vi "test_read-nmea-data2.vi"() -> ()   [LabVIEW 2019] (continued)
15:15:18.22\tF9P\t\t\n15:15:18.24\tF9P\t$GNRMC,061520.00,A,3723.59873,N,12656.93743,E,2.458,246.74,250720,,,A,V*09\n\t\n15:15:18.26\tF9P\t$GNVTG,246.74,T,,M,2.458,N,4.552,K,A*2D\n\t\n15:15:18.28\tF9P\t$GNGGA,061520.00,3723.59873,N,12656.93743,E,1,12,0.71,46.1,M,18.5,M,,*71\n\t\n15:15:18.30\tF9P\t$GNGSA,A,3,12,06,19,05,17,09,04,02,,,,,1.21,0.71,0.98,1*05\n\t\n15:15:18.32\tF9P\t$GNGSA,A,3,85,70,71,84,,,,,,,,,1.21,0.71,0.98,2*07\n\t\n15:15:18.34\tF9P\t$GNGSA,A,3,36,19,11,04,09,12,,,,,,,1.21,0.71,0.98,3*05\n\t\n15:15:18.36\tF9P\t$GNGSA,A,3,14,11,33,,,,,,,,,,1.21,0.71,0.98,4*04\n\t\n15:15:18.38\tF9P\t$GPGSV,3,1,09,02,56,320,31,04,17,043,28,05,38,248,31,06,64,051,27,1*65\n\t\n15:15:18.40\tF9P\t$GPGSV,3,2,09,09,44,072,41,12,23,275,26,17,31,154,27,19,51,157,28,1*67\n\t\n15:15:18.42\tF9P\t$GPGSV,3,3,09,25,12,305,21,1*5C\n\t\n15:15:18.44\tF9P\t$GPGSV,3,1,09,02,56,320,,04,17,043,22,05,38,248,31,06,64,051,29,6*64\n\t\n15:15:18.46\tF9P\t$GPGSV,3,2,09,09,44,072,34,12,23,275,18,17,31,154,20,19,51,157,,6*62\n\t\n15:15:18.48\tF9P\t$GPGSV,3,3,09,25,12,305,,6*58\n\t\n15:15:18.50\tF9P\t$GLGSV,2,1,08,69,10,031,27,70,70,037,28,71,54,207,33,72,05,210,,1*75\n\t\n15:15:18.52\tF9P\t$GLGSV,2,2,08,77,01,324,,84,19,123,16,85,69,072,38,86,38,331,,1*7F\n\t\n15:15:18.54\tF9P\t$GLGSV,2,1,08,69,10,031,20,70,70,037,,71,54,207,24,72,05,210,,3*7C\n\t\n15:15:18.56\tF9P\t$GLGSV,2,2,08,77,01,324,,84,19,123,20,85,69,072,26,86,38,331,,3*77\n\t\n15:15:18.58\tF9P\t$GAGSV,2,1,08,02,08,296,11,04,67,114,38,09,33,193,29,11,72,001,24,7*7E\n\t\n15:15:18.60\tF9P\t$GAGSV,2,2,08,12,39,103,24,19,25,045,30,25,08,248,,36,27,309,22,7*70\n\t\n15:15:18.62\tF9P\t$GAGSV,2,1,08,02,08,296,,04,67,114,,09,33,193,21,11,72,001,,2*7E\n\t\n15:15:18.64\tF9P\t$GAGSV,2,2,08,12,39,103,,19,25,045,22,25,08,248,,36,27,309,19,2*78\n\t\n15:15:18.66\tF9P\t$GBGSV,2,1,06,07,,,24,11,48,133,27,14,87,101,28,28,,,26,1*74\n\t\n15:15:18.68\tF9P\t$GBGSV,2,2,06,33,62,220,32,34,,,32,1*43\n\t\n15:15:18.70\tF9P\t$GBGSV,1,1,03,11,48,133,25,14,87,101,29,33,62,220,,3*48\n\t\n15:15:18.72\tF9P\t$GNGLL,3723.59873,N,12656.93743,E,061520.00,A,A*7E\n\t\n15:15:18.74\tF9P\t\t\n15:15:18.76\tF9P\t\t\n15:15:18.78\tF9P\t\t\n15:15:18.80\tF9P\t\t\n15:15:18.82\tF9P\t\t\n15:15:18.84\tF9P\t\t\n15:15:18.86\tF9P\t\t\n15:15:18.88\tF9P\t\t\n15:15:18.90\tF9P\t\t\n15:15:18.92\tF9P\t\t\n15:15:18.94\tF9P\t\t\n15:15:18.96\tF9P\t\t\n15:15:18.98\tF9P\t\t\n15:15:19.00\tF9P\t\t\n15:15:19.02\tF9P\t\t\n15:15:19.04\tF9P\t\t\n15:15:19.06\tF9P\t\t\n15:15:19.08\tF9P\t\t\n15:15:19.10\tF9P\t\t\n15:15:19.12\tF9P\t\t\n15:15:19.14\tF9P\t\t\n15:15:19.16\tF9P\t\t\n15:15:19.18\tF9P\t\t\n15:15:19.20\tF9P\t\t\n15:15:19.22\tF9P\t\t\n15:15:19.24\tF9P\t$GNRMC,061521.00,A,3723.59850,N,12656.93661,E,2.546,240.41,250720,,,A,V*06\n\t\n15:15:19.26\tF9P\t$GNVTG,240.41,T,,M,2.546,N,4.715,K,A*22\n\t\n15:15:19.28\tF9P\t$GNGGA,061521.00,3723.59850,N,12656.93661,E,1,12,0.68,46.5,M,18.5,M,,*7C\n\t\n15:15:19.30\tF9P\t$GNGSA,A,3,12,06,19,05,17,09,04,02,,,,,1.19,0.68,0.98,1*06\n\t\n15:15:19.32\tF9P\t$GNGSA,A,3,85,70,71,84,,,,,,,,,1.19,0.68,0.98,2*04\n\t\n15:15:19.34\tF9P\t$GNGSA,A,3,36,19,11,04,09,12,,,,,,,1.19,0.68,0.98,3*06\n\t\n15:15:19.36\tF9P\t$GNGSA,A,3,14,11,33,,,,,,,,,,1.19,0.68,0.98,4*07\n\t\n15:15:19.38\tF9P\t$GPGSV,3,1,09,02,56,320,25,04,17,043,27,05,38,248,30,06,64,051,26,1*6F\n\t\n15:15:19.40\tF9P\t$GPGSV,3,2,09,09,44,072,43,12,23,275,35,17,31,154,28,19,51,157,28,1*68\n\t\n15:15:19.42\tF9P\t$GPGSV,3,3,09,25,12,305,20,1*5D\n\t\n15:15:19.44\tF9P\t$GPGSV,3,1,09,02,56,320,,04,17,043,21,05,38,248,22,06,64,051,29,6*65\n\t\n15:15:19.46\tF9P\t$GPGSV,3,2,09,09,44,072,31,12,23,275,18,17,31,154,18,19,51,157,,6*6C\n\t\n15:15:19.48\tF9P\t$GPGSV,3,3,09,25,12,305,,6*58\n\t\n15:15:19.50\tF9P\t$GLGSV,2,1,08,69,10,031,25,70,70,037,29,71,54,207,37,72,05,210,,1*72\n\t\n15:15:19.52\tF9P\t$GLGSV,2,2,08,77,01,324,,84,19,123,14,85,69,072,37,86,38,331,,1*72\n\t\n15:15:19.54\tF9P\t$GLGSV,2,1,08,69,10,031,19,70,70,037,,71,54,207,25,72,05,210,,3*77\n\t\n15:15:19.56\tF9P\t$GLGSV,2,2,08,77,01,324,,84,19,123,20,85,69,072,26,86,38,331,,3*77\n\t\n15:15:19.58\tF9P\t$GAGSV,2,1,08,02,08,296,10,04,67,114,39,09,33,193,35,11,72,001,24,7*73\n\t\n15:15:19.60\tF9P\t$GAGSV,2,2,08,12,39,103,24,19,25,045,28,25,08,248,,36,27,309,23,7*78\n\t\n15:15:19.62\tF9P\t$GAGSV,2,1,08,02,08,296,,04,67,114,,09,33,193,20,11,72,001,,2*7F\n\t\n15:15:19.64\tF9P\t$GAGSV,2,2,08,12,39,103,,19,25,045,22,25,08,248,,36,27,309,18,2*79\n\t\n15:15:19.66\tF9P\t$GBGSV,2,1,06,07,,,24,11,48,133,28,14,87,101,32,28,,,26,1*70\n\t\n15:15:19.68\tF9P\t$GBGSV,2,2,06,33,62,220,33,34,,,26,1*47\n\t\n15:15:19.70\tF9P\t$GBGSV,1,1,03,11,48,133,,14,87,101,,33,62,220,,3*44\n\t\n15:15:19.72\tF9P\t$GNGLL,3723.59850,N,12656.93661,E,061521.00,A,A*7F\n\t\n15:15:19.74\tF9P\t\t\n15:15:19.76\tF9P\t\t\n15:15:19.78\tF9P\t\t\n15:15:19.80\tF9P\t\t\n15:15:19.82\tF9P\t\t\n15:15:19.84\tF9P\t\t\n15:15:19.86\tF9P\t\t\n15:15:19.88\tF9P\t\t\n15:15:19.90\tF9P\t\t\n15:15:19.92\tF9P\t\t\n15:15:19.94\tF9P\t\t\n15:15:19.96\tF9P\t\t\n15:15:19.98\tF9P\t\t\n15:15:20.00\tF9P\t\t\n15:15:20.02\tF9P\t\t\n15:15:20.04\tF9P\t\t\n15:15:20.06\tF9P\t\t\n15:15:20.08\tF9P\t\t\n15:15:20.10\tF9P\t\t\n15:15:20.12\tF9P\t\t\n15:15:20.14\tF9P\t\t\n15:15:20.16\tF9P\t\t\n15:15:20.18\tF9P\t\t\n15:15:20.20\tF9P\t\t\n15:15:20.22\tF9P\t\t\n15:15:20.24\tF9P\t$GNRMC,061522.00,A,3723.59832,N,12656.93567,E,2.630,241.81,250720,,,A,V*0B\n\t\n15:15:20.26\tF9P\t$GNVTG,241.81,T,,M,2.630,N,4.870,K,A*21\n\t\n15:15:20.28\tF9P\t$GNGGA,061522.00,3723.59832,N,12656.93567,E,1,12,0.65,46.4,M,18.5,M,,*72\n\t\n15:15:20.30\tF9P\t$GNGSA,A,3,12,06,19,05,17,09,04,02,,,,,1.15,0.65,0.95,1*0A\n\t\n15:15:20.32\tF9P\t$GNGSA,A,3,85,70,71,84,,,,,,,,,1.15,0.65,0.95,2*08\n\t\n15:15:20.34\tF9P\t$GNGSA,A,3,36,19,11,04,09,12,,,,,,,1.15,0.65,0.95,3*0A\n\t\n15:15:20.36\tF9P\t$GNGSA,A,3,14,11,33,,,,,,,,,,1.15,0.65,0.95,4*0B\n\t\n15:15:20.38\tF9P\t$GPGSV,3,1,09,02,56,320,31,04,17,043,38,05,38,248,29,06,64,051,31,1*6A\n\t\n15:15:20.40\tF9P\t$GPGSV,3,2,09,09,44,072,40,12,23,275,32,17,31,154,29,19,51,157,28,1*6D\n\t\n15:15:20.42\tF9P\t$GPGSV,3,3,09,25,12,305,19,1*57\n\t\n15:15:20.44\tF9P\t$GPGSV,3,1,09,02,56,320,,04,17,043,21,05,38,248,22,06,64,051,28,6*64\n\t\n15:15:20.46\tF9P\t$GPGSV,3,2,09,09,44,072,26,12,23,275,18,17,31,154,19,19,51,157,,6*6B\n\t\n15:15:20.48\tF9P\t$GPGSV,3,3,09,25,12,305,,6*58\n\t\n15:15:20.50\tF9P\t$GLGSV,2,1,08,69,10,031,25,70,70,037,24,71,54,207,29,72,05,210,,1*70\n\t\n15:15:20.52\tF9P\t$GLGSV,2,2,08,77,01,324,,84,19,123,14,85,69,072,35,86,38,331,,1*70\n\t\n15:15:20.54\tF9P\t$GLGSV,2,1,08,69,10,031,18,70,70,037,,71,54,207,30,72,05,210,,3*72\n\t\n15:15:20.56\tF9P\t$GLGSV,2,2,08,77,01,324,,84,19,123,20,85,69,072,26,86,38,331,,3*77\n\t\n15:15:20.58\tF9P\t$GAGSV,2,1,08,02,08,296,13,04,67,114,36,09,33,193,26,11,72,001,25,7*7C\n\t\n15:15:20.60\tF9P\t$GAGSV,2,2,08,12,39,103,25,19,25,045,29,25,08,248,,36,27,309,23,7*78\n\t\n15:15:20.62\tF9P\t$GAGSV,2,1,08,02,08,296,,04,67,114,,09,33,193,20,11,72,001,,2*7F\n\t\n15:15:20.64\tF9P\t$GAGSV,2,2,08,12,39,103,,19,25,045,21,25,08,248,,36,27,309,20,2*71\n\t\n15:15:20.66\tF9P\t$GBGSV,2,1,06,07,,,29,11,48,133,26,14,87,101,29,28,,,25,1*7A\n\t\n15:15:20.68\tF9P\t$GBGSV,2,2,06,33,62,220,38,34,,,25,1*4F\n\t\n15:15:20.70\tF9P\t$GBGSV,1,1,03,11,48,133,,14,87,101,,33,62,220,,3*44\n\t\n15:15:20.72\tF9P\t$GNGLL,3723.59832,N,12656.93567,E,061522.00,A,A*7D\n\t\n15:15:20.74\tF9P\t\t\n15:15:20.76\tF9P\t\t\n15:15:20.78\tF9P\t\t\n15:15:20.80\tF9P\t\t\n15:15:20.82\tF9P\t\t\n15:15:20.84\tF9P\t\t\n15:15:20.86\tF9P\t\t\n15:15:20.88\tF9P\t\t\n15:15:20.90\tF9P\t\t\n15:15:20.92\tF9P\t\t\n15:15:20.94\tF9P\t\t\n15:15:20.96\tF9P\t\t\n15:15:20.98\tF9P\t\t\n15:15:21.00\tF9P\t\t\n15:15:21.02\tF9P\t\t\n15:15:21.04\tF9P\t\t\n15:15:21.06\tF9P\t\t\n15:15:21.08\tF9P\t\t\n15:15:21.10\tF9P\t\t\n15:15:21.12\tF9P\t\t\n15:15:21.14\tF9P\t\t\n15:15:21.16\tF9P\t\t\n15:15:21.18\tF9P\t\t\n15:15:21.20\tF9P\t\t\n15:15:21.22\tF9P\t\t\n15:15:21.24\tF9P\t$GNRMC,061523.00,A,3723.59801,N,12656.93492,E,2.349,237.20,250720,,,A,V*00\n\t\n15:15:21.26\tF9P\t$GNVTG,237.20,T,,M,2.349,N,4.350,K,A*29\n\t\n15:15:21.29\tF9P\t$GNGGA,061523.00,3723.59801,N,12656.93492,E,1,12,0.69,46.6,M,18.5,M,,*76\n\t\n15:15:21.31\tF9P\t$GNGSA,A,3,12,06,19,05,17,09,04,02,,,,,1.20,0.69,0.98,1*0D\n\t\n15:15:21.33\tF9P\t$GNGSA,A,3,85,70,71,84,,,,,,,,,1.20,0.69,0.98,2*0F\n\t\n15:15:21.35\tF9P\t$GNGSA,A,3,36,19,11,04,09,12,,,,,,,1.20,0.69,0.98,3*0D\n\t\n15:15:21.37\tF9P\t$GNGSA,A,3,14,11,33,,,,,,,,,,1.20,0.69,0.98,4*0C\n\t\n15:15:21.39\tF9P\t$GPGSV,3,1,09,02,56,320,25,04,17,043,35,05,38,248,31,06,64,051,31,1*6B\n\t\n15:15:21.41\tF9P\t$GPGSV,3,2,09,09,44,072,42,12,23,275,31,17,31,154,28,19,51,157,27,1*62\n\t\n15:15:21.43\tF9P\t$GPGSV,3,3,09,25,12,305,18,1*56\n\t\n15:15:21.45\tF9P\t$GPGSV,3,1,09,02,56,320,,04,17,043,20,05,38,248,21,06,64,051,28,6*66\n\t\n15:15:21.47\tF9P\t$GPGSV,3,2,09,09,44,072,31,12,23,275,20,17,31,154,18,19,51,157,,6*67\n\t\n15:15:21.49\tF9P\t$GPGSV,3,3,09,25,12,305,,6*58\n\t\n15:15:21.51\tF9P\t$GLGSV,2,1,08,69,10,031,31,70,70,037,30,71,54,207,31,72,05,210,,1*79\n\t\n15:15:21.53\tF9P\t$GLGSV,2,2,08,77,01,324,,84,19,123,15,85,69,072,38,86,38,331,,1*7C\n\t\n15:15:21.55\tF9P\t$GLGSV,2,1,08,69,10,031,18,70,70,037,,71,54,207,24,72,05,210,,3*77\n\t\n15:15:21.57\tF9P\t$GLGSV,2,2,08,77,01,324,,84,19,123,21,85,69,072,25,86,38,331,,3*75\n\t\n15:15:21.59\tF9P\t$GAGSV,2,1,08,02,08,296,15,04,67,114,32,09,33,193,27,11,72,001,24,7*7E\n\t\n15:15:21.61\tF9P\t$GAGSV,2,2,08,12,39,103,26,19,25,045,29,25,08,248,,36,27,309,23,7*7B\n\t\n15:15:21.63\tF9P\t$GAGSV,2,1,08,02,08,296,,04,67,114,,09,33,193,22,11,72,001,,2*7D\n\t\n15:15:21.65\tF9P\t$GAGSV,2,2,08,12,39,103,,19,25,045,21,25,08,248,,36,27,309,,2*73\n\t\n15:15:21.67\tF9P\t$GBGSV,2,1,06,07,,,24,11,48,133,27,14,87,101,37,28,,,25,1*79\n\t\n15:15:21.69\tF9P\t$GBGSV,2,2,06,33,62,220,38,34,,,24,1*4E\n\t\n15:15:21.71\tF9P\t$GBGSV,1,1,03,11,48,133,,14,87,101,,33,62,220,,3*44\n\t\n15:15:21.73\tF9P\t$GNGLL,3723.59801,N,12656.93492,E,061523.00,A,A*77\n\t\n15:15:21.75\tF9P\t\t\n15:15:21.77\tF9P\t\t\n15:15:21.79\tF9P\t\t\n15:15:21.81\tF9P\t\t\n15:15:21.83\tF9P\t\t\n15:15:21.85\tF9P\t\t\n15:15:21.87\tF9P\t\t\n15:15:21.89\tF9P\t\t\n15:15:21.91\tF9P\t\t\n15:15:21.93\tF9P\t\t\n15:15:21.95\tF9P\t\t\n15:15:21.97\tF9P\t\t\n15:15:21.99\tF9P\t\t\n15:15:22.01\tF9P\t\t\n15:15:22.03\tF9P\t\t\n15:15:22.05\tF9P\t\t\n15:15:22.07\tF9P\t\t\n15:15:22.09\tF9P\t\t\n15:15:22.11\tF9P\t\t\n15:15:22.13\tF9P\t\t\n15:15:22.15\tF9P\t\t\n15:15:22.17\tF9P\t\t\n15:15:22.19\tF9P\t\t\n15:15:22.21\tF9P\t\t\n15:15:22.23\tF9P\t$GNRMC,061524.00,A,3723.59778,N,12656.93396,E,2.598,237.74,250720,,,A,V*0E\n\t\n15:15:22.25\tF9P\t$GNVTG,237.74,T,,M,2.598,N,4.811,K,A*2C\n\t\n15:15:22.27\tF9P\t$GNGGA,061524.00,3723.59778,N,12656.93396,E,1,12,0.71,46.5,M,18.5,M,,*79\n\t\n15:15:22.29\tF9P\t$GNGSA,A,3,12,06,19,05,17,09,04,02,,,,,1.21,0.71,0.98,1*05\n\t\n15:15:22.31\tF9P\t$GNGSA,A,3,85,70,71,84,,,,,,,,,1.21,0.71,0.98,2*07\n\t\n15:15:22.33\tF9P\t$GNGSA,A,3,36,19,11,04,09,12,,,,,,,1.21,0.71,0.98,3*05\n\t\n15:15:22.35\tF9P\t$GNGSA,A,3,14,11,33,,,,,,,,,,1.21,0.71,0.98,4*04\n\t\n15:15:22.37\tF9P\t$GPGSV,3,1,09,02,56,320,31,04,17,043,27,05,38,248,30,06,64,051,36,1*6B\n\t\n15:15:22.39\tF9P\t$GPGSV,3,2,09,09,44,072,26,12,23,275,36,17,31,154,26,19,51,157,27,1*69\n\t\n15:15:22.41\tF9P\t$GPGSV,3,3,09,25,12,305,19,1*57\n\t\n15:15:22.43\tF9P\t$GPGSV,3,1,09,02,56,320,,04,17,043,20,05,38,248,21,06,64,051,27,6*69\n\t\n15:15:22.45\tF9P\t$GPGSV,3,2,09,09,44,072,26,12,23,275,28,17,31,154,17,19,51,157,,6*66\n\t\n15:15:22.47\tF9P\t$GPGSV,3,3,09,25,12,305,,6*58\n\t\n15:15:22.49\tF9P\t$GLGSV,2,1,08,69,10,031,25,70,70,037,25,71,54,207,31,72,05,210,,1*78\n\t\n15:15:22.51\tF9P\t$GLGSV,2,2,08,77,01,324,,84,19,123,15,85,69,072,36,86,38,331,,1*72\n\t\n15:15:22.53\tF9P\t$GLGSV,2,1,08,69,10,031,17,70,70,037,,71,54,207,24,72,05,210,,3*78\n\t\n15:15:22.55\tF9P\t$GLGSV,2,2,08,77,01,324,,84,19,123,21,85,69,072,31,86,38,331,,3*70\n\t\n15:15:22.57\tF9P\t$GAGSV,2,1,08,02,08,296,11,04,67,114,35,09,33,193,27,11,72,002,25,7*7F\n\t\n15:15:22.59\tF9P\t$GAGSV,2,2,08,12,39,103,25,19,25,045,33,25,08,248,,36,27,309,27,7*77\n\t\n15:15:22.61\tF9P\t$GAGSV,2,1,08,02,08,296,,04,67,114,,09,33,193,30,11,72,002,,2*7D\n\t\n15:15:22.63\tF9P\t$GAGSV,2,2,08,12,39,103,,19,25,045,22,25,08,248,,36,27,309,,2*70\n\t\n15:15:22.65\tF9P\t$GBGSV,2,1,06,07,,,23,11,48,133,40,14,87,101,38,28,,,25,1*70\n\t\n15:15:22.67\tF9P\t$GBGSV,2,2,06,33,62,220,35,34,,,31,1*47\n\t\n15:15:22.69\tF9P\t$GBGSV,1,1,03,11,48,133,,14,87,101,,33,62,220,,3*44\n\t\n15:15:22.71\tF9P\t$GNGLL,3723.59778,N,12656.93396,E,061524.00,A,A*72\n\t\n15:15:22.73\tF9P\t\t\n15:15:22.75\tF9P\t\t\n15:15:22.77\tF9P\t\t\n15:15:22.79\tF9P\t\t\n15:15:22.81\tF9P\t\t\n15:15:22.83\tF9P\t\t\n15:15:22.85\tF9P\t\t\n15:15:22.87\tF9P\t\t\n15:15:22.89\tF9P\t\t\n15:15:22.91\tF9P\t\t\n15:15:22.93\tF9P\t\t\n15:15:22.95\tF9P\t\t\n15:15:22.97\tF9P\t\t\n15:15:22.99\tF9P\t\t\n15:15:23.01\tF9P\t\t\n15:15:23.03\tF9P\t\t\n15:15:23.05\tF9P\t\t\n15:15:23.07\tF9P\t\t\n15:15:23.09\tF9P\t\t\n15:15:23.11\tF9P\t\t\n15:15:23.13\tF9P\t\t\n15:15:23.15\tF9P\t\t\n15:15:23.17\tF9P\t\t\n15:15:23.19\tF9P\t\t\n15:15:23.21\tF9P\t\t\n15:15:23.23\tF9P\t$GNRMC,061525.00,A,3723.59752,N,12656.93310,E,2.415,240.50,250720,,,A,V*0B\n\t\n15:15:23.25\tF9P\t$GNVTG,240.50,T,,M,2.415,N,4.473,K,A*26\n\t\n15:15:23.27\tF9P\t$GNGGA,061525.00,3723.59752,N,12656.93310,E,1,12,0.76,46.8,M,18.5,M,,*74\n\t\n15:15:23.29\tF9P\t$GNGSA,A,3,12,06,19,05,17,09,04,02,,,,,1.26,0.76,1.01,1*04\n\t\n15:15:23.31\tF9P\t$GNGSA,A,3,85,70,71,84,,,,,,,,,1.26,0.76,1.01,2*06\n\t\n15:15:23.33\tF9P\t$GNGSA,A,3,36,19,11,04,09,12,,,,,,,1.26,0.76,1.01,3*04\n\t\n15:15:23.35\tF9P\t$GNGSA,A,3,14,11,33,,,,,,,,,,1.26,0.76,1.01,4*05\n\t\n15:15:23.37\tF9P\t$GPGSV,3,1,09,02,56,320,30,04,17,043,26,05,38,248,23,06,64,051,34,1*6B\n\t\n15:15:23.39\tF9P\t$GPGSV,3,2,09,09,44,072,32,12,23,275,32,17,31,154,26,19,51,157,27,1*68\n\t\n15:15:23.41\tF9P\t$GPGSV,3,3,09,25,12,305,19,1*57\n\t\n15:15:23.43\tF9P\t$GPGSV,3,1,09,02,56,320,,04,17,043,20,05,38,248,21,06,64,051,26,6*68\n\t\n15:15:23.45\tF9P\t$GPGSV,3,2,09,09,44,072,26,12,23,275,27,17,31,154,16,19,51,157,,6*68\n\t\n15:15:23.47\tF9P\t$GPGSV,3,3,09,25,12,305,,6*58\n\t\n15:15:23.49\tF9P\t$GLGSV,2,1,08,69,10,031,24,70,70,037,25,71,54,207,37,72,05,210,,1*7F\n\t\n15:15:23.51\tF9P\t$GLGSV,2,2,08,77,01,324,,84,19,123,13,85,69,072,28,86,38,331,,1*7B\n\t\n15:15:23.53\tF9P\t$GLGSV,2,1,08,69,10,031,16,70,70,037,,71,54,207,30,72,05,210,,3*7C\n\t\n15:15:23.55\tF9P\t$GLGSV,2,2,08,77,01,324,,84,19,123,20,85,69,072,22,86,38,331,,3*73\n\t\n15:15:23.57\tF9P\t$GAGSV,2,1,08,02,08,296,07,04,67,114,39,09,33,193,27,11,72,002,24,7*75\n\t\n15:15:23.59\tF9P\t$GAGSV,2,2,08,12,39,104,24,19,25,045,29,25,08,248,,36,27,309,24,7*79\n\t\n15:15:23.61\tF9P\t$GAGSV,2,1,08,02,08,296,,04,67,114,,09,33,193,,11,72,002,,2*7E\n\t\n15:15:23.63\tF9P\t$GAGSV,2,2,08,12,39,104,,19,25,045,,25,08,248,,36,27,309,,2*77\n\t\n15:15:23.65\tF9P\t$GBGSV,2,1,06,07,,,25,11,48,133,32,14,87,101,35,28,,,27,1*7C\n\t\n15:15:23.67\tF9P\t$GBGSV,2,2,06,33,62,220,31,34,,,24,1*47\n\t\n15:15:23.69\tF9P\t$GBGSV,1,1,03,11,48,133,,14,87,101,26,33,62,220,,3*40\n\t\n15:15:23.71\tF9P\t$GNGLL,3723.59752,N,12656.93310,E,061525.00,A,A*75\n\t\n15:15:23.73\tF9P\t\t\n15:15:23.75\tF9P\t\t\n15:15:23.77\tF9P\t\t\n15:15:23.79\tF9P\t\t\n15:15:23.81\tF9P\t\t\n15:15:23.83\tF9P\t\t\n15:15:23.85\tF9P\t\t\n15:15:23.87\tF9P\t\t\n15:15:23.89\tF9P\t\t\n15:15:23.91\tF9P\t\t\n15:15:23.93\tF9P\t\t\n15:15:23.95\tF9P\t\t\n15:15:23.97\tF9P\t\t\n15:15:23.99\tF9P\t\t\n15:15:24.01\tF9P\t\t\n15:15:24.03\tF9P\t\t\n15:15:24.05\tF9P\t\t\n15:15:24.07\tF9P\t\t\n15:15:24.09\tF9P\t\t\n15:15:24.11\tF9P\t\t\n15:15:24.13\tF9P\t\t\n15:15:24.15\tF9P\t\t\n15:15:24.17\tF9P\t\t\n15:15:24.19\tF9P\t\t\n15:15:24.21\tF9P\t\t\n15:15:24.23\tF9P\t$GNRMC,061526.00,A,3723.59745,N,12656.93258,E,0.975,242.83,250720,,,A,V*06\n\t\n15:15:24.25\tF9P\t$GNVTG,242.83,T,,M,0.975,N,1.806,K,A*28\n\t\n15:15:24.27\tF9P\t$GNGGA,061526.00,3723.59745,N,12656.93258,E,1,12,0.77,46.9,M,18.5,M,,*7C\n\t\n15:15:24.29\tF9P\t$GNGSA,A,3,12,06,19,05,17,09,04,02,,,,,1.26,0.77,1.00,1*04\n\t\n15:15:24.31\tF9P\t$GNGSA,A,3,85,70,71,84,,,,,,,,,1.26,0.77,1.00,2*06\n\t\n15:15:24.33\tF9P\t$GNGSA,A,3,36,19,11,04,09,12,,,,,,,1.26,0.77,1.00,3*04\n\t\n15:15:24.35\tF9P\t$GNGSA,A,3,14,11,33,,,,,,,,,,1.26,0.77,1.00,4*05\n\t\n15:15:24.37\tF9P\t$GPGSV,3,1,09,02,56,320,25,04,17,043,,05,38,248,25,06,64,051,35,1*6C\n\t\n15:15:24.39\tF9P\t$GPGSV,3,2,09,09,44,072,28,12,23,275,29,17,31,154,17,19,51,157,28,1*64\n\t\n15:15:24.41\tF9P\t$GPGSV,3,3,09,25,12,305,18,1*56\n\t\n15:15:24.43\tF9P\t$GPGSV,3,1,09,02,56,320,,04,17,043,20,05,38,248,21,06,64,051,26,6*68\n\t\n15:15:24.45\tF9P\t$GPGSV,3,2,09,09,44,072,25,12,23,275,27,17,31,154,15,19,51,157,,6*68\n\t\n15:15:24.47\tF9P\t$GPGSV,3,3,09,25,12,305,,6*58\n\t\n15:15:24.49\tF9P\t$GLGSV,2,1,08,69,10,031,23,70,70,037,25,71,54,207,36,72,05,210,,1*79\n\t\n15:15:24.51\tF9P\t$GLGSV,2,2,08,77,01,324,,84,19,123,13,85,69,072,34,86,38,331,,1*76\n\t\n15:15:24.53\tF9P\t$GLGSV,2,1,08,69,10,031,16,70,70,037,,71,54,207,31,72,05,210,,3*7D\n\t\n15:15:24.55\tF9P\t$GLGSV,2,2,08,77,01,324,,84,19,123,19,85,69,072,22,86,38,331,,3*79\n\t\n15:15:24.57\tF9P\t$GAGSV,2,1,08,02,08,296,13,04,67,114,37,09,33,193,33,11,72,002,26,7*79\n\t\n15:15:24.59\tF9P\t$GAGSV,2,2,08,12,39,104,25,19,25,045,22,25,08,248,,36,27,309,24,7*73\n\t\n15:15:24.61\tF9P\t$GAGSV,2,1,08,02,08,296,,04,67,114,30,09,33,193,,11,72,002,,2*7D\n\t\n15:15:24.63\tF9P\t$GAGSV,2,2,08,12,39,104,,19,25,045,,25,08,248,,36,27,309,,2*77\n\t\n15:15:24.65\tF9P\t$GBGSV,2,1,06,07,,,24,11,48,133,27,14,87,101,33,28,,,29,1*71\n\t\n15:15:24.67\tF9P\t$GBGSV,2,2,06,33,62,220,41,34,,,30,1*45\n\t\n15:15:24.69\tF9P\t$GBGSV,1,1,03,11,48,133,,14,87,101,33,33,62,220,,3*44\n\t\n15:15:24.71\tF9P\t$GNGLL,3723.59745,N,12656.93258,E,061526.00,A,A*7D\n\t\n15:15:24.73\tF9P\t\t\n15:15:24.75\tF9P\t\t\n15:15:24.77\tF9P\t\t\n15:15:24.79\tF9P\t\t\n15:15:24.81\tF9P\t\t\n15:15:24.83\tF9P\t\t\n15:15:24.85\tF9P\t\t\n15:15:24.87\tF9P\t\t\n15:15:24.89\tF9P\t\t\n15:15:24.91\tF9P\t\t\n15:15:24.93\tF9P\t\t\n15:15:24.95\tF9P\t\t\n15:15:24.97\tF9P\t\t\n15:15:24.99\tF9P\t\t\n15:15:25.01\tF9P\t\t\n15:15:25.03\tF9P\t\t\n15:15:25.05\tF9P\t\t\n15:15:25.07\tF9P\t\t\n15:15:25.09\tF9P\t\t\n15:15:25.11\tF9P\t\t\n15:15:25.13\tF9P\t\t\n15:15:25.15\tF9P\t\t\n15:15:25.17\tF9P\t\t\n15:15:25.19\tF9P\t\t\n15:15:25.21\tF9P\t\t\n15:15:25.23\tF9P\t$GNRMC,061527.00,A,3723.59755,N,12656.93215,E,0.121,,250720,,,A,V*17\n\t\n15:15:25.25\tF9P\t$GNVTG,,T,,M,0.121,N,0.224,K,A*3B\n\t\n15:15:25.27\tF9P\t$GNGGA,061527.00,3723.59755,N,12656.93215,E,1,12,0.77,46.3,M,18.5,M,,*7F\n\t\n15:15:25.29\tF9P\t$GNGSA,A,3,12,06,19,05,17,09,04,02,,,,,1.26,0.77,1.00,1*04\n\t\n15:15:25.31\tF9P\t$GNGSA,A,3,85,70,71,84,,,,,,,,,1.26,0.77,1.00,2*06\n\t\n15:15:25.33\tF9P\t$GNGSA,A,3,36,19,11,04,09,12,,,,,,,1.26,0.77,1.00,3*04\n\t\n15:15:25.35\tF9P\t$GNGSA,A,3,14,11,33,,,,,,,,,,1.26,0.77,1.00,4*05\n\t\n15:15:25.37\tF9P\t$GPGSV,3,1,09,02,56,320,24,04,17,043,33,05,38,248,34,06,64,051,29,1*60\n\t\n15:15:25.39\tF9P\t$GPGSV,3,2,09,09,44,072,39,12,23,275,41,17,31,154,27,19,51,157,28,1*69\n\t\n15:15:25.41\tF9P\t$GPGSV,3,3,09,25,12,305,19,1*57\n\t\n15:15:25.43\tF9P\t$GPGSV,3,1,09,02,56,320,,04,17,043,19,05,38,248,22,06,64,051,32,6*64\n\t\n15:15:25.45\tF9P\t$GPGSV,3,2,09,09,44,072,25,12,23,275,25,17,31,154,14,19,51,157,,6*6B\n\t\n15:15:25.47\tF9P\t$GPGSV,3,3,09,25,12,305,,6*58\n\t\n15:15:25.49\tF9P\t$GLGSV,2,1,08,69,10,031,24,70,70,037,24,71,54,207,37,72,05,210,,1*7E\n\t\n15:15:25.51\tF9P\t$GLGSV,2,2,08,77,01,324,,84,19,123,15,85,69,072,35,86,38,331,,1*71\n\t\n15:15:25.53\tF9P\t$GLGSV,2,1,08,69,10,031,15,70,70,037,,71,54,207,25,72,05,210,,3*7B\n\t\n15:15:25.55\tF9P\t$GLGSV,2,2,08,77,01,324,,84,19,123,16,85,69,072,23,86,38,331,,3*77\n\t\n15:15:25.57\tF9P\t$GAGSV,2,1,08,02,08,296,11,04,67,114,37,09,33,193,29,11,72,002,32,7*75\n\t\n15:15:25.59\tF9P\t$GAGSV,2,2,08,12,39,104,25,19,25,045,26,25,08,248,,36,27,309,21,7*72\n\t\n15:15:25.61\tF9P\t$GAGSV,2,1,08,02,08,296,,04,67,114,24,09,33,193,,11,72,002,,2*78\n\t\n15:15:25.63\tF9P\t$GAGSV,2,2,08,12,39,
